vi "Capture@CallVI__Parameter.vi"(1 "ParamterIn":string) -> (0 "ParamterOut":string)   [LabVIEW 2019]
uses:
  MainFrame/Global.vi
panel:
  in  "Parameters":string(combo)
  in  "VI":string(combo)
  in  "Confirm":bool
  # "User@CallVI $VI,$Parameter"
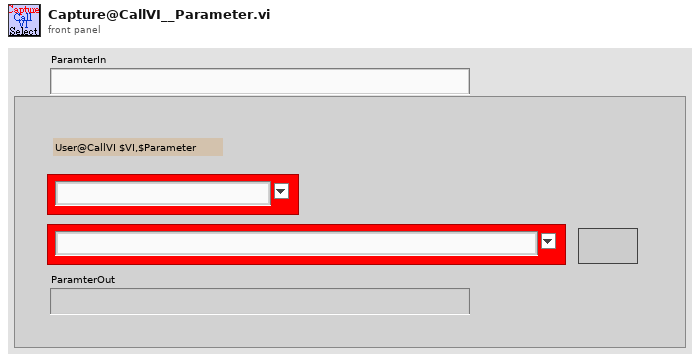
[diagram p1: front panel]
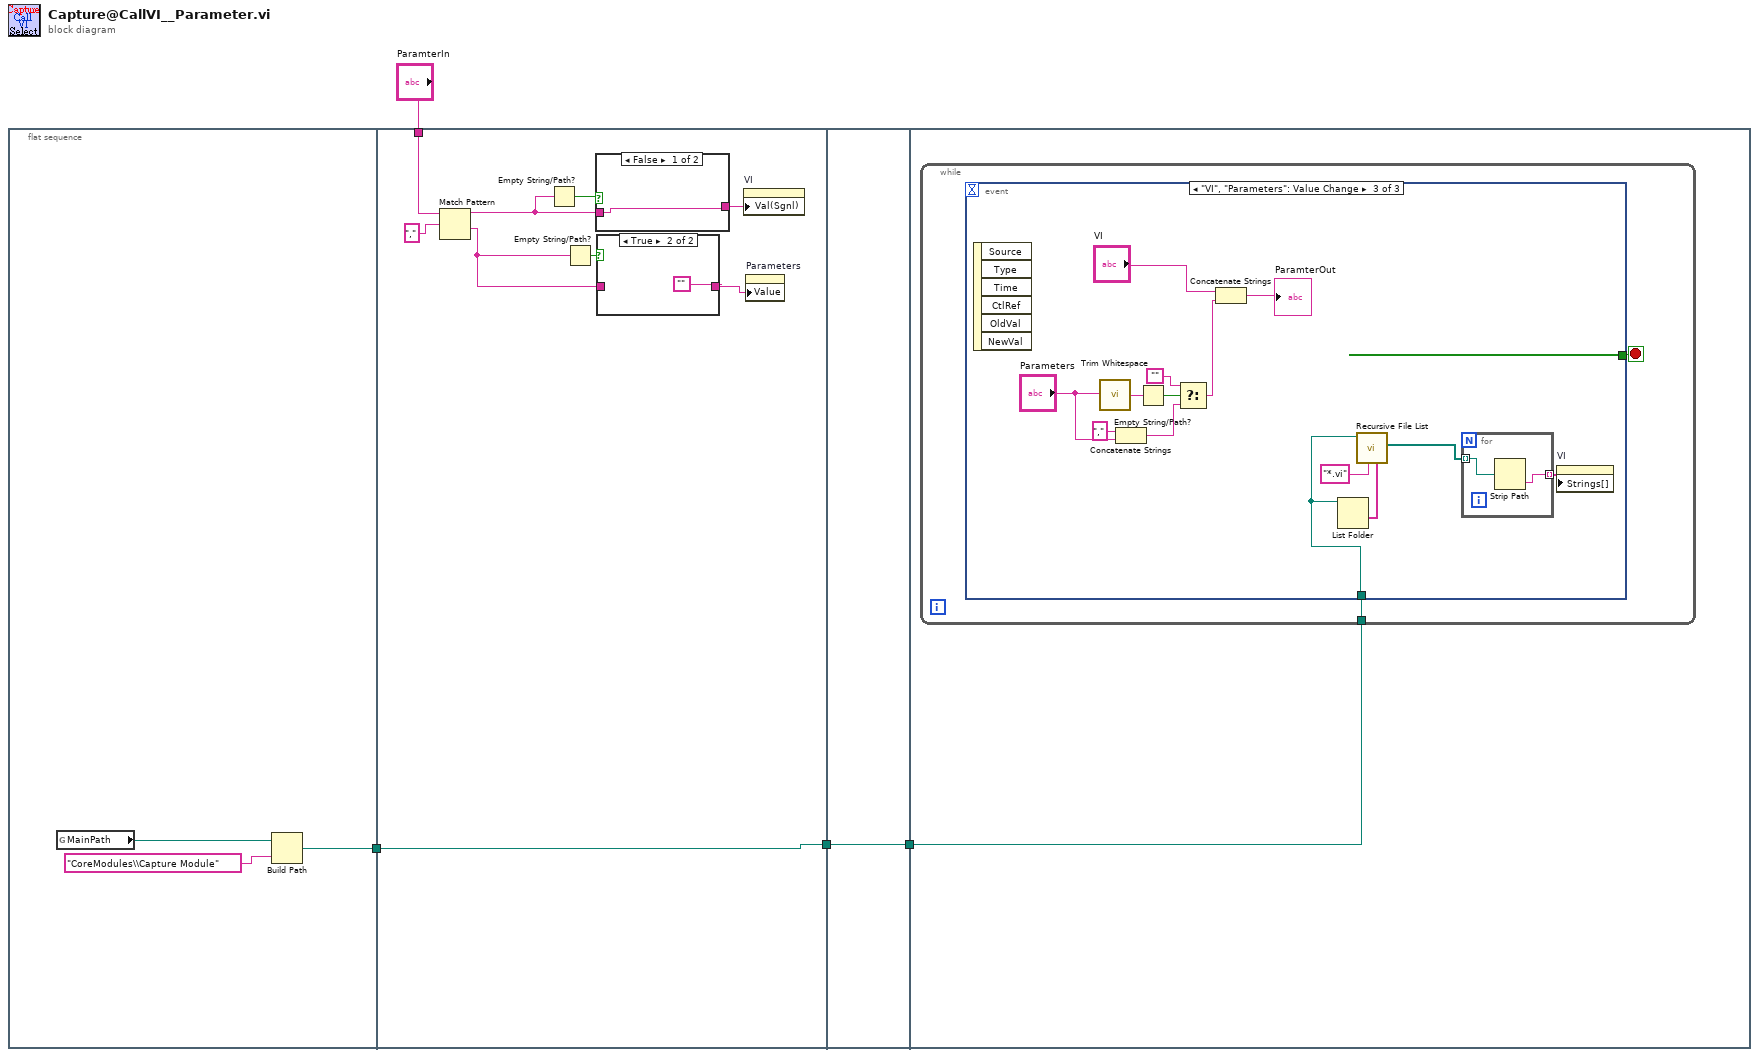
[diagram p0: block diagram]
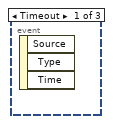
[diagram p4: hidden frame]
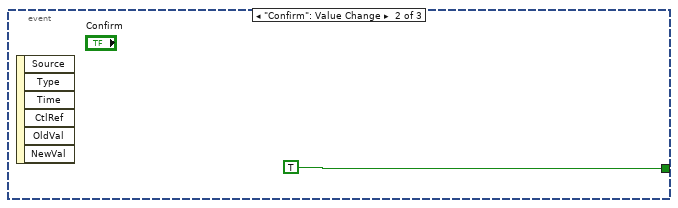
[diagram p5: hidden frame]
diagram:
  n1 = flat-sequence {
    tunnel: [w6] -> w1
    tunnel: "ParamterIn" -> [w13]
    tunnel: [w14] -> w2
    tunnel: w1 -> [w14]
    tunnel: [w21] -> w3
    tunnel: w2 -> [w21]
    tunnel: w3 -> [w22]
    frame #0 {
      n2 = global read "Global.vi" "MainPath"() -> (w5:path)
      n3 = Build Path(base path=w5, name or relative path="CoreModules\\Capture Module") -> (appended path=w6:path)
    }
    frame #1 {
      n4 = Match Pattern(string=w13, regular expression=",") -> (before substring=w11:string, after substring=w10:string)  [unwired: 1 in, 2 out]
      n5 = Empty String/Path?(string/path=w11) -> (empty?=w16:bool)
      n6 = Empty String/Path?(string/path=w10) -> (empty?=w15:bool)
      n7 = case shown="False" w16 {
        tunnel: w11 -> [w19 w20]
        tunnel: [w19 w20] -> w8
        frame False {
        }
        frame True {
        }
      }
      n8 = case shown="True" w15 {
        tunnel: [w17 ""] -> w9
        tunnel: w10 -> [w17 _]
        frame False {
        }
        frame True {
        }
      }
      n9 = property on="VI" class="CmbBox"("Val(Sgnl)"=w8) -> ()  [unwired: 2 in, 2 out]
      n10 = property on="Parameters" class="CmbBox"("Value"=w9) -> ()  [unwired: 2 in, 2 out]
    }
    frame #2 {
    }
    frame #3 {
      n11 = while {
        tunnel: w22 -> [w23]
        stop <- w24 stop-if-true
        n12 = event shown="[2] \"VI\", \"Parameters\": Value Change" {
          selector: _ -> [_ _ _]
          dyn-events: _ -> [_ _ _]
          timeout: _ -> [_ _ _]
          tunnel: [_ TRUE _] -> w24
          tunnel: w23 -> [_ _ w27]
          event Timeout {
            n13 = event-data() -> ()  [unwired: 1 in, 3 out]
          }
          event "Confirm": Value Change {
            n14 = event-data() -> ()  [unwired: 1 in, 6 out]
          }
          event "VI", "Parameters": Value Change {
            n15 = event-data() -> ()  [unwired: 1 in, 6 out]
            n16 = call <vilib>:"Trim Whitespace.vi"("string"="Parameters") -> ("trimmed string"=w33:string)  [unwired: 1 in]
            n17 = Concatenate Strings("," ("string"), "Parameters") -> (w32:string)
            n18 = Empty String/Path?(string/path=w33) -> (empty?=w34:bool)
            n19 = Select(t="", s=w34, f=w32) -> (s? t:f=w28:string)
            n20 = Concatenate Strings("VI", w28) -> (→"ParamterOut":string)
            n21 = List Folder(path=w27) -> (folder names=w26:string[])  [unwired: 3 in, 3 out]
            n22 = call <vilib>:"Recursive File List.vi"("Folders to Exclude"=w26, "pattern"="*.vi", "Folder Path"=w27) -> ("All Files in Dir"=w37:path[])  [unwired: 4 in, 4 out]
            n23 = for {
              tunnel: w37 -> [w41] mode=indexing
              tunnel: [w40] -> w29 mode=indexing
              n24 = Strip Path(path=w41) -> (name=w40:string)  [unwired: 1 out]
            }
            n25 = property on="VI" class="CmbBox"("Strings[]"=w29) -> ()  [unwired: 2 in, 2 out]
          }
        }
      }
    }
  }
